vi "Get Number Missed External Triggers.vi"(7 "size":u32, 8 "error in (no error)":errorcluster, 9 "arr":u16, 10 "last":u32, 11 "first":u32) -> (0 "error out":errorcluster, 1 "arr out":u16, 3 "function return":u32)   [LabVIEW 2014, in "atmcd32d.lvlib"]
doc: "unsigned int WINAPI GetNumberMissedExternalTriggers(unsigned int first, unsigned int last, WORD * arr, unsigned int size);"
uses:
  atmcd32d.lvlib
  atmcd32d.dll
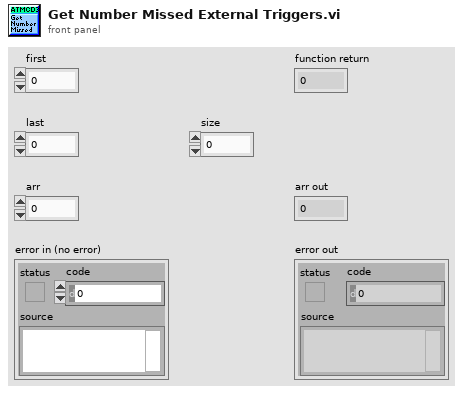
[diagram p1: front panel]
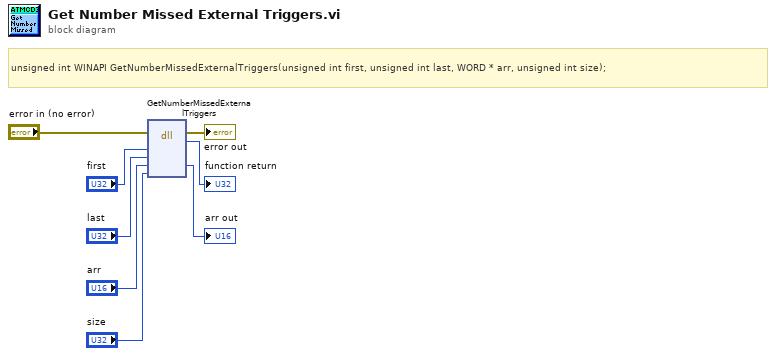
[diagram p0: block diagram]
diagram:
  # "unsigned int WINAPI GetNumberMissedExternalTriggers(unsigned int first, unsigned int last, WORD * arr, unsigned int size);"
  n1 = dll-call lib="C:/Users/Bakir/Documents/Lambda2-Testing/lib/Andorlib/atmcd32d.*" fn="GetNumberMissedExternalTriggers"(error in="error in (no error)", "first"="first", "last"="last", "arr"="arr", "size"="size") -> (error out=→"error out":errorcluster, →"function return":u32, "arr"=→"arr out":u16)  [unwired: 5 in, 1 out]
